vi "Generate write queue item.vi"(8 "error in (no error)":errorcluster, 10 "Request ID":u64, 11 "Publish JSON in":refnum<class "Publish JSON.lvclass">) -> (0 "error out":errorcluster, 2 "Write queue item":T1, 3 "Publish JSON out":refnum<class "Publish JSON.lvclass">)   [LabVIEW 2020, in "wamplv.lvlib" / "Publish JSON.lvclass"]
uses:
  Publish JSON.lvclass
  Publish JSON.lvclass/Publish JSON.ctl
  TypeDefs/WAMP Message Codes.ctl
  wamplv.lvlib
  Utils/Utils.lvclass
  <vilib>/JDP Science/JSONtext/JSONtext.lvlib
  2c5b81e0-7822-4892-9d8a-f1863cf115ca.vi
  TypeDefs/Transport type.ctl
  WAMP Client/Private/TypeDef/Write queue item.ctl
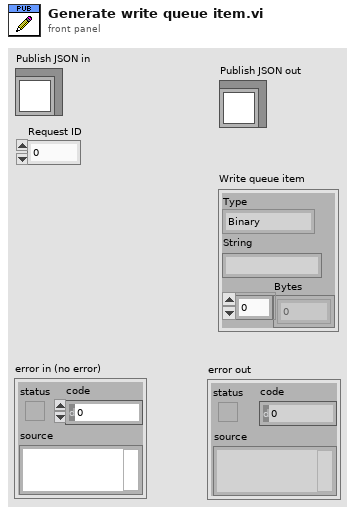
[diagram p1: front panel]
types:
  T1 = typedef "wamplv.lvlib/Write queue item.ctl" = cluster{"Type":T2, "String":string, "Bytes":u8[]}
  T2 = typedef "wamplv.lvlib/Transport type.ctl" = enum16{"Binary", "Text"}
  T3 = typedef "wamplv.lvlib/WAMP Message Codes.ctl" = enum8{"HELLO", "WELCOME", "CHALLENGE", "AUTHENTICATE", "ABORT", "GOODBYE", "ERROR", "PUBLISH", "PUBLISHED", "SUBSCRIBE", "SUBSCRIBED", "UNSUBSCRIBE", "UNSUBSCRIBED", "EVENT", "CALL", "RESULT", "REGISTER", "REGISTERED", "UNREGISTER", "UNREGISTERED", "INVOCATION", "YIELD"}
  T4 = typedef "wamplv.lvlib/PUBLISH Request Data (JSON).ctl" = cluster{"Topic URI":string, "Arguments":string, "ArgumentsKw":string, "Request Acknowledgement":bool, "Options":string, "Publish result notifier":refnum<notifier>}
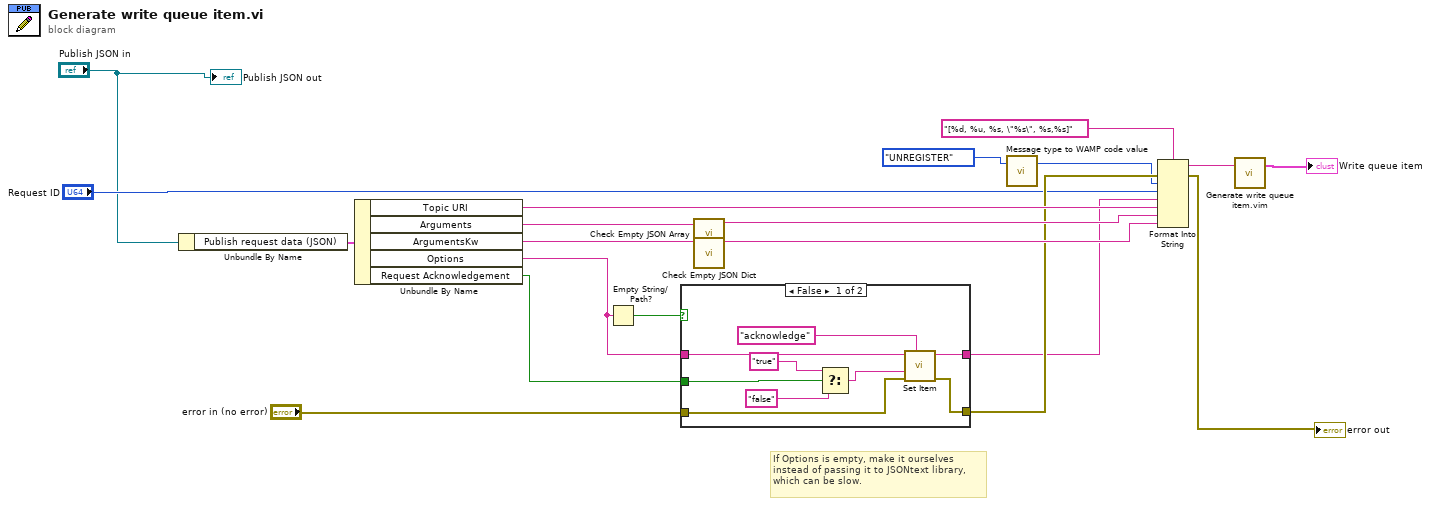
[diagram p0: block diagram]
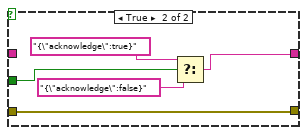
[diagram p2: hidden frame]
diagram:
  # "If Options is empty, make it ourselves \ninstead of passing it to JSONtext library, \nwhich can be slow."
  n1 = Unbundle By Name("Publish JSON in") -> ("Publish request data (JSON)"=w2:T4)
  n2 = Unbundle By Name(w2) -> ("Topic URI"=w19:string, "Arguments"=w16:string, "ArgumentsKw"=w18:string, "Options"=w11:string, "Request Acknowledgement"=w10:bool)
  n3 = Empty String/Path?(string/path=w11) -> (empty?=w12:bool)
  n4 = case shown="False" w12 {
    tunnel: [w28 w32] -> w14
    tunnel: "error in (no error)" -> [w27 w32]
    tunnel: [w26 w31] -> w13
    tunnel: w11 -> [w25 _]
    tunnel: w10 -> [w21 w30]
    frame False {
      n5 = Select(t="true" ("JSON to Insert"), s=w21, f="false") -> (s? t:f=w22:string)
      n6 = call <vilib>:"Set Item.vi"("$Path or Item Name"="acknowledge", "error in (no error)"=w27, "JSON to Insert"=w22, "JSON"=w25) -> ("error out"=w28:errorcluster, "<JSON>"=w26:string)  [unwired: 4 in, 1 out]
    }
    frame True {
      n7 = Select(t="{\"acknowledge\":true}" ("JSON to Insert"), s=w30, f="{\"acknowledge\":false}") -> (s? t:f=w31:string)
    }
  }
  n8 = call "Check Empty JSON Array.vi"("JSON in"=w16) -> ("JSON out"=w15:string)  [unwired: 10 in]
  n9 = call "Check Empty JSON Dict.vi"("JSON in"=w18) -> ("JSON out"=w17:string)  [unwired: 10 in]
  n10 = call "Message type to WAMP code value.vi"("Message Type"=WAMP_Message_Codes."UNREGISTER" ("Message Codes")) -> ("WAMP Numeric value"=w3:u8)  [unwired: 2 in]
  n11 = Format Into String(format string="[%d, %u, %s, \"%s\", %s,%s]" ("element"), error in=w14, w3, "Request ID", w13, w19, w15, w17) -> (resulting string=w6:string, error out=→"error out":errorcluster)  [unwired: 1 in]
  n12 = call "Generate write queue item.vim"("Input"=w6) -> ("Ouput"=→"Write queue item":T1)  [unwired: 2 in]
  "Publish JSON out" <- "Publish JSON in"
